vi "ClientSignature.vi"(8 "error in (no error)":errorcluster, 9 "Authenticate Extra  Data":T1, 10 "Challenge data":T2, 11 "WampScramAuthenticator in":refnum<class "WampScramAuthenticator.lvclass">) -> (0 "error out":errorcluster, 2 "Client Signature":u8[](array[numeric]), 3 "WampScramAuthenticator out":refnum<class "WampScramAuthenticator.lvclass">)   [LabVIEW 2020, in "wamplv.lvlib" / "WampScramAuthenticator.lvclass"]
uses:
  WampScramAuthenticator.lvclass
  WampScramAuthenticator.lvclass/WampScramAuthenticator.ctl
  HashLib/HashLib.lvclass
  Utils/Utils.lvclass
  TypeDefs/Challenge data.ctl
  TypeDefs/Authenticate Extra data.ctl
  TypeDefs/HMAC parameters.ctl
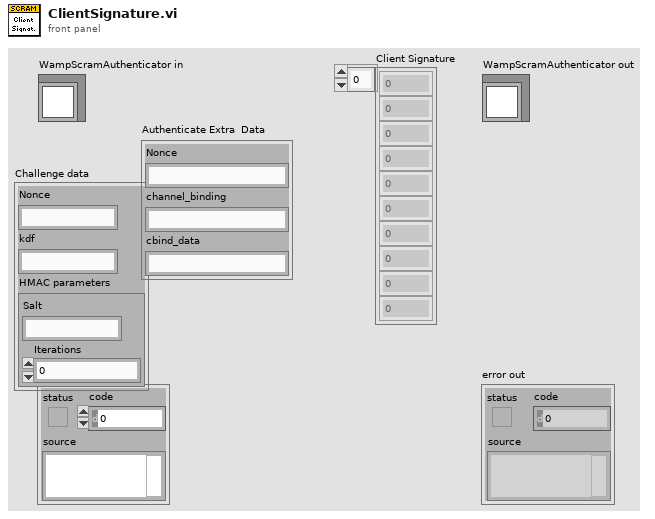
[diagram p1: front panel]
types:
  T1 = typedef "wamplv.lvlib/WampScramAuthenticator.lvclass/Authenticate Extra data.ctl" = cluster{"Nonce":string, "channel_binding":string, "cbind_data":string}
  T2 = typedef "wamplv.lvlib/WampScramAuthenticator.lvclass/Challenge data.ctl" = cluster{"Nonce":string, "kdf":string, "HMAC parameters":T3}
  T3 = typedef "wamplv.lvlib/WampScramAuthenticator.lvclass/HMAC parameters.ctl" = cluster{"Salt":string, "Iterations":i32}
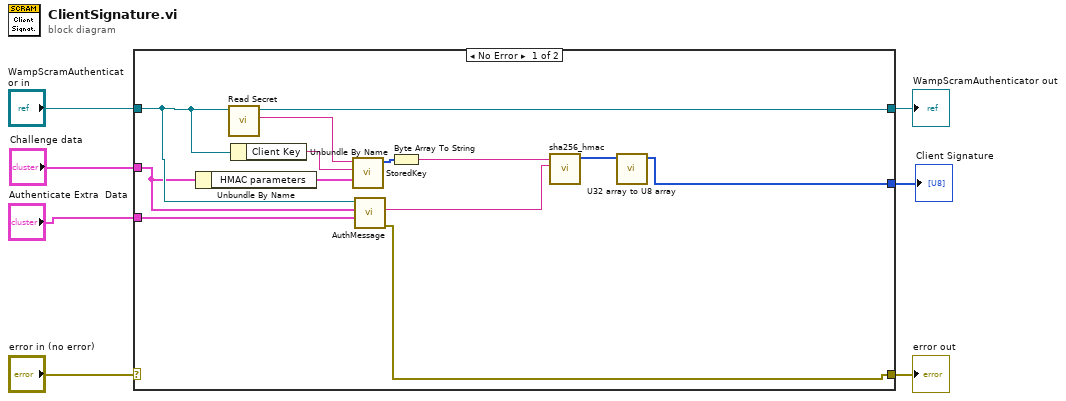
[diagram p0: block diagram]
diagram:
  n1 = case shown="No Error" "error in (no error)" {
    selector: "error in (no error)" -> [_ w22]
    tunnel: [w14 w22] -> w6
    tunnel: [w13 w21] -> w4
    tunnel: "WampScramAuthenticator in" -> [w11 w21]
    tunnel: "Challenge data" -> [w9 _]
    tunnel: "Authenticate Extra  Data" -> [w18 _]
    tunnel: [w16 _] -> w1
    frame No Error {
      n2 = Unbundle By Name(w9) -> ("HMAC parameters"=w8:T3)
      n3 = call-dynamic "Read Secret.vi"("SecretBasedAuthenticatorBase in"=w11) -> ("Secret"=w12:string, "SecretBasedAuthenticatorBase out"=w13:refnum<class "WampScramAuthenticator.lvclass">)  [unwired: 8 in, 1 out]
      n4 = Unbundle By Name(w11) -> ("Client Key"=w10:string)
      n5 = call "StoredKey.vi"("HMAC parameters"=w8, "Un-hashed client Key"=w10, "Secret"=w12) -> ("StoredKey"=w15:u8[])  [unwired: 8 in]
      n6 = call "AuthMessage.vi"("Authenticate Extra  Data"=w18, "Challenge data"=w9, "WampScramAuthenticator in"=w11) -> ("error out"=w14:errorcluster, "AuthMessage"=w20:string)  [unwired: 6 in, 1 out]
      n7 = Byte Array To String(unsigned byte array=w15) -> (string=w19:string)
      n8 = call "sha256_hmac.vi"("data"=w20, "key"=w19) -> ("sha256"=w17:u32[])  [unwired: 9 in]
      n9 = call "U32 array to U8 array.vi"("Array in"=w17) -> ("Array out"=w16:u8[])  [unwired: 10 in]
    }
    frame Error {
    }
  }
  "error out" <- w6
  "WampScramAuthenticator out" <- w4
  "Client Signature" <- w1
